vi "超标留样启动命令.vi"() -> (0 "error out":errorcluster)   [LabVIEW 2016, in "超标留样集成.lvlib"]
uses:
  DR803M4/DR803M4.lvlib
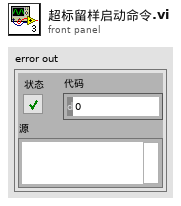
[diagram p1: front panel]
types:
  T1 = enum16{"德润DR803M", "德润DR803L", "德润DR803F", "科盛超标留样", "德润DR803M4"}
  T2 = cluster{"STEP":enum16{"open", "read", "write", "close"}, "写入缓冲区":string}
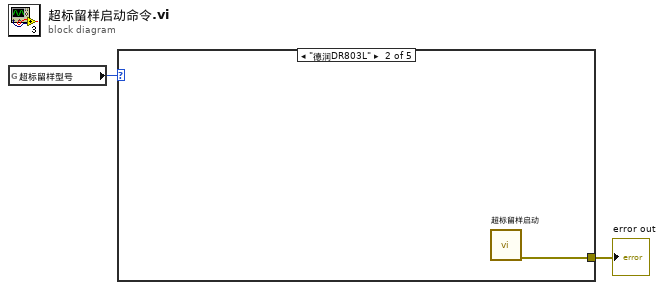
[diagram p0: block diagram]
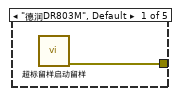
[diagram p2: hidden frame]
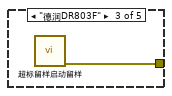
[diagram p3: hidden frame]
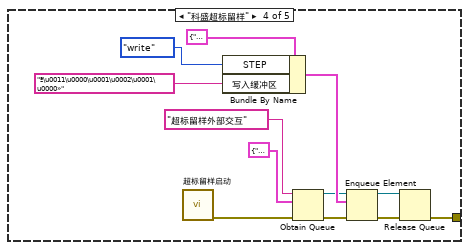
[diagram p4: hidden frame]
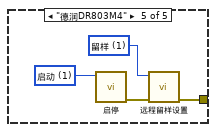
[diagram p5: hidden frame]
diagram:
  n1 = global read "断电保存全局.vi" "超标留样型号"() -> (w2:T1)
  n2 = case shown="\"德润DR803L\"" w2 {
    tunnel: [w3 w4 w5 w6 w18] -> w1
    frame "德润DR803M", Default {
      n3 = call "超标留样启动留样.vi"() -> ("error out"=w3:errorcluster)  [unwired: 11 in]
    }
    frame "德润DR803L" {
      n4 = call "超标留样启动.vi"() -> ("error out"=w4:errorcluster)  [unwired: 11 in]
    }
    frame "德润DR803F" {
      n5 = call "超标留样启动留样.vi"() -> ("error out"=w5:errorcluster)  [unwired: 11 in]
    }
    frame "科盛超标留样" {
      n6 = call "超标留样启动.vi"() -> ("error out"=w9:errorcluster)  [unwired: 11 in]
      n7 = Bundle By Name(cluster=T2 {"STEP"=enum."open", "写入缓冲区"=""} ("元素"), "STEP"=enum16{"open", "read", "write", "close"}."write", "写入缓冲区"="ª\u0011\u0000\u0001\u0002\u0001\u0000»") -> (w13:T2)
      n8 = Obtain Queue(name (unnamed)="超标留样外部交互" ("名称（未命名）"), element data type=T2 {"STEP"=enum."write", "写入缓冲区"="ª\u0006\u0000\u0000P`\u00000»"}, error in (no error)=w9) -> (queue out=w11:refnum<queue>, error out=w10:errorcluster)  [unwired: 2 in, 1 out]
      n9 = Enqueue Element(queue=w11, element=w13, error in (no error)=w10) -> (queue out=w7:refnum<queue>, error out=w8:errorcluster)  [unwired: 1 in, 1 out]
      n10 = Release Queue(queue=w7, error in (no error)=w8) -> (error out=w6:errorcluster)  [unwired: 1 in, 2 out]
    }
    frame "德润DR803M4" {
      w20 = u16 1 items=["停止", "留样"] ("远程留样")
      w21 = u16 1 items=["停止", "启动"] ("启停")
      n11 = call "启停.vi"("启停"=w21) -> ("error out"=w19:errorcluster)  [unwired: 10 in]
      n12 = call "远程留样设置.vi"("error in (no error)"=w19, "远程留样"=w20) -> ("error out"=w18:errorcluster)  [unwired: 9 in]
    }
  }
  "error out" <- w1
